vi "main.vi"() -> ()   [LabVIEW 2014]
uses:
  Kimematics Param.ctl
  <vilib>/Platform/TimedLoop/XDataNode/timing_clust.ctl
  <vilib>/Platform/TimedLoop/XDataNode/nitl_modes.ctl
  <vilib>/Platform/TimedLoop/XDataNode/wakeup.ctl
  <vilib>/Platform/TimedLoop/XDataNode/loadnilvce.vi
  <vilib>/Motion/Express/_s/nimc.fb.write.writeSetpoint.axis.vi
  <vilib>/platform/TimedLoop/XDataNode/XDataNode.xnode
  <vilib>/Motion/BlockNode/FB.NIMotion.xnode
  <vilib>/Platform/TimedLoop/XDataNode/XDNodeRunTimeDep.lvlib
panel:
  out "error in":errorcluster
  out "inRange":bool
  out "Debug":dbl[](array[numeric])
  in  "stop":bool
  out "Axis 3":dbl(slide) scale=400.0..-30.0
  out "Axis 2":dbl(slide) scale=400.0..-30.0
  out "Axis 1":dbl(slide) scale=400.0..-30.0
  in  "Y":dbl(slide) scale=-60.0..60.0
  in  "X":dbl(slide) scale=-60.0..60.0
  in  "Z":dbl(slide) scale=55.0..30.0
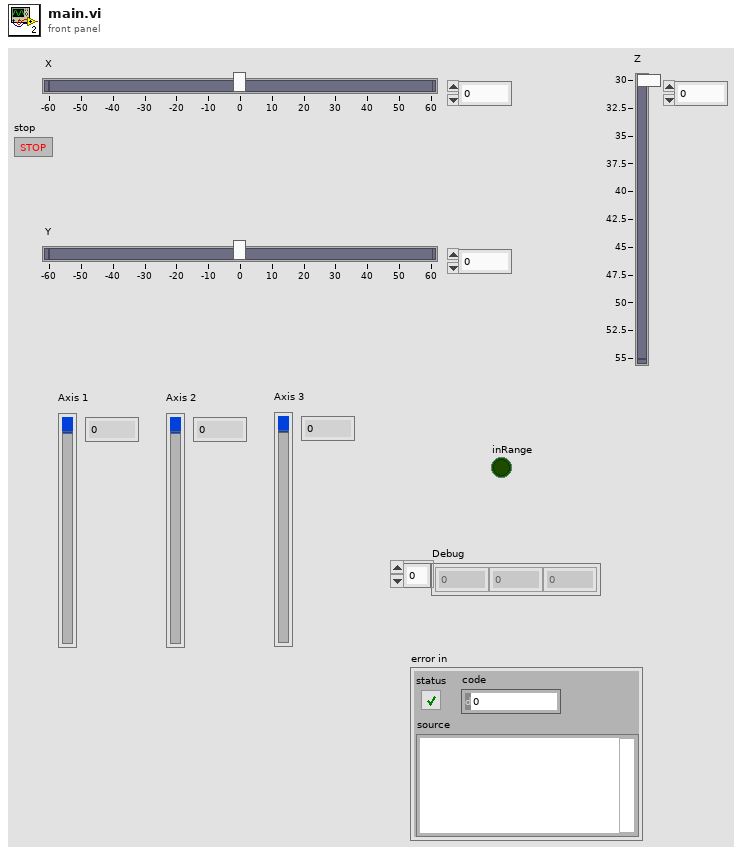
[diagram p1: front panel]
types:
  T1 = typedef "Kimematics Param.ctl" = cluster{"Length of arms \"a\" (cm)":dbl, "Length of arms \"b\" (cm)":dbl, "Length of  base \"r\" (cm)":dbl, "Length of platform \"h\" (cm)":dbl, "Phi (deg)":dbl[], "Upper limit of Theta":dbl, "Lower limit of Theta":dbl}
  T2 = typedef "XDNodeRunTimeDep.lvlib/timing_clust.ctl" = cluster{"Expected End [f-1]":u64, "Actual End [f-1]":u64, "Finished Late? [f-1]":bool, "Expected End [i-1]":u64, "Actual End [i-1]":u64, "Finished Late? [i-1]":bool, "Expected Start [i]":u64, "Actual Start [i]":u64, "Expected Start [f]":u64, "Actual Start [f]":u64, "Source Name":string, "Structure Name":string, "Period":i64, "Deadline":i64, "Offset":i64, "Start":i64, "Priority":i32, "Timeout":i32, "Mode":T3, "Wakeup Reason":T4, "Error":errorcluster, "Source Type":string, "Secondary Source Type":string, "Global End Time":u64, "Global Start Time":u64, "Frame Duration":u64, "Iteration Duration":u64, "Assigned CPU":i32, "I/O Scan Engine Mode":u32}
  T3 = typedef "XDNodeRunTimeDep.lvlib/nitl_modes.ctl" = enum32{"No Change", "Process missed periods, maintain original phase", "Discard missed periods, maintain original phase", "Process missed periods, ignore original phase", "Discard missed periods, ignore original phase"}
  T4 = typedef "XDNodeRunTimeDep.lvlib/wakeup.ctl" = enum32{"Normal", "Aborted", "Asynchronous wakeup", "Timing source error", "Timed loop error", "Timeout"}
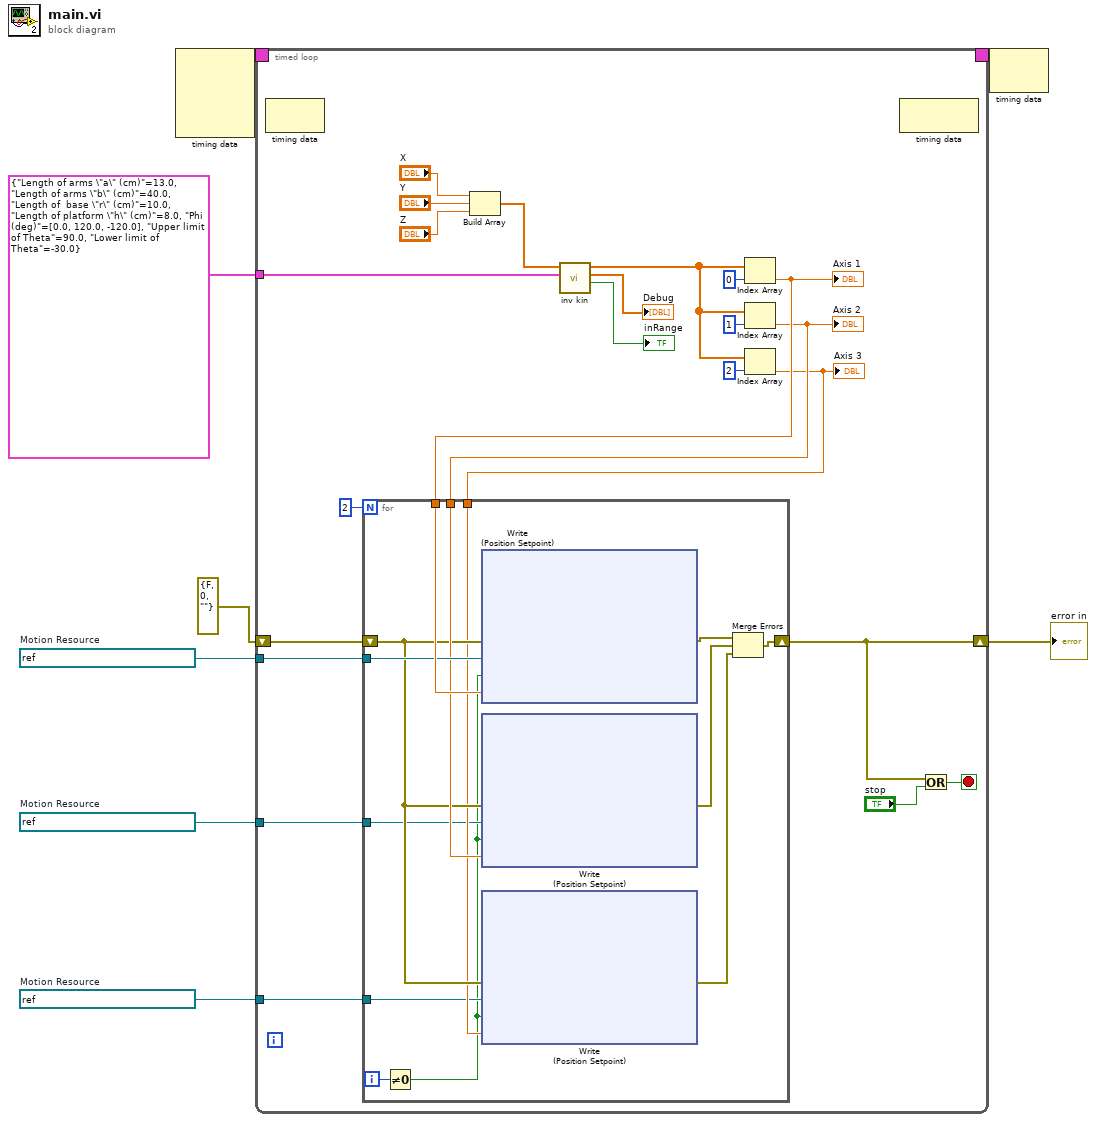
[diagram p0: block diagram]
diagram:
  w3 = refnum<k21> "nism://My Computer/Axis 3"  # Motion Resource
  w4 = refnum<k21> "nism://My Computer/Axis 2"  # Motion Resource
  w5 = refnum<k21> "nism://My Computer/Axis 1"  # Motion Resource
  n1 = node-c288() -> (w8:T2)  [unwired: 4 in]
  n2 = timed-loop {
    timing: w8 -> [_]
    timing-out: [_] -> w7
    shift-right: [w17] -> w1
    shift-left: errorcluster {"status"=FALSE, "code"=0, "source"=""} ("error in") -> [w21]
    tunnel: w5 -> [w19]
    tunnel: w4 -> [w14]
    tunnel: w3 -> [w13]
    tunnel: T1 {"Length of arms \"a\" (cm)"=13.0, "Length of arms \"b\" (cm)"=40.0, "Length of  base \"r\" (cm)"=10.0, "Length of platform \"h\" (cm)"=8.0, "Phi (deg)"=[0.0, 120.0, -120.0], "Upper limit of Theta"=90.0, "Lower limit of Theta"=-30.0} ("Kinematics Param") -> [w9]
    stop <- w23 stop-if-true
    n3 = node-c288() -> ()  [unwired: 1 in, 1 out]
    n4 = Build Array("X", "Y", "Z") -> (w27:dbl[])
    n5 = call "inv kin.vi"("Kinematics Param"=w9, "Point of TCF (X,Y,Z)"=w27) -> ("inRange"=→"inRange":bool, "Debug"=→"Debug":dbl[], "Theta (deg)"=w12:dbl[])  [unwired: 7 in]
    n6 = Index Array(array=w12, index=0) -> (element=w20:dbl)
    "Axis 1" <- w20
    n7 = Index Array(array=w12, index=1) -> (element=w16:dbl)
    "Axis 2" <- w16
    n8 = Index Array(array=w12, index=2) -> (element=w15:dbl)
    "Axis 3" <- w15
    n9 = for {
      N: 2 -> [_]
      tunnel: w20 -> [w43]
      tunnel: w19 -> [w41]
      shift-right: [w40] -> w17
      shift-left: w21 -> [w35]
      tunnel: w16 -> [w38]
      tunnel: w15 -> [w34]
      tunnel: w14 -> [w33]
      tunnel: w13 -> [w32]
      i -> [w42]
      n10 = Not Equal To 0?(x=w42) -> (x != 0?=w31:bool)
      n11 = xnode "Write\n(Position Setpoint)"("error in"=w35, "resource"=w41, "execute"=w31, "position setpoint"=w43) -> ("error out"=w39:errorcluster)  [unwired: 2 out]
      n12 = xnode "Write\n(Position Setpoint)"("error in"=w35, "resource"=w33, "execute"=w31, "position setpoint"=w38) -> ("error out"=w37:errorcluster)  [unwired: 2 out]
      n13 = xnode "Write\n(Position Setpoint)"("error in"=w35, "resource"=w32, "execute"=w31, "position setpoint"=w34) -> ("error out"=w36:errorcluster)  [unwired: 2 out]
      n14 = Merge Errors(w39, w37, w36) -> (w40:errorcluster)
    }
    n15 = node-c288() -> ()  [unwired: 1 in, 1 out]
    n16 = Or(x=w17, y="stop") -> (x .or. y?=w23:bool)
  }
  "error in" <- w1
  n17 = node-c288(w7) -> ()  [unwired: 1 out]
